vi "DUAL GAUGE-Watchdog control.vi"(7 "W/R":bool, 8 "Fehler (Eingang)":errorcluster, 9 "Watchdog Set":u8(ring) items=["off", "on"], 11 "Referenz in":refnum<visa-resource-name>) -> (0 "Cluster (Ausgang)":errorcluster, 1 "Watchdog Get":u8(ring) items=["off", "on"], 3 "Referenz out":refnum<visa-resource-name>)   [LabVIEW 2013, in "Dual Gauge.lvlib"]
uses:
  Dual Gauge.lvlib
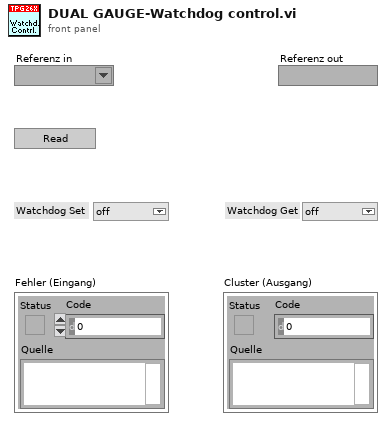
[diagram p1: front panel]
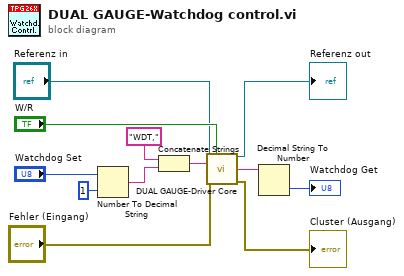
[diagram p0: block diagram]
diagram:
  n1 = Number To Decimal String(number="Watchdog Set", width (-)=i16 1) -> (decimal integer string=w6:string)
  n2 = Concatenate Strings("WDT,", w6) -> (w5:string)
  n3 = call "DUAL GAUGE-Driver Core.vi"("Referenz in"="Referenz in", "Write/Read"="W/R", "Command"=w5, "Fehler (Eingang)"="Fehler (Eingang)") -> ("Referenz out"=→"Referenz out":refnum<visa-resource-name>, "String Out"=w8:string, "Cluster (Ausgang)"=→"Cluster (Ausgang)":errorcluster)  [unwired: 9 in]
  n4 = Decimal String To Number(string=w8) -> (number=→"Watchdog Get":i32)  [unwired: 2 in, 1 out]
